vi "关键参数区.vi"(11 "数组":u16[](array[numeric]) format="%04xH") -> (3 "关键参数区":T1)   [LabVIEW 2016, in "CODCr库.lvlib"]
panel:
  # "共占用56 WORD"
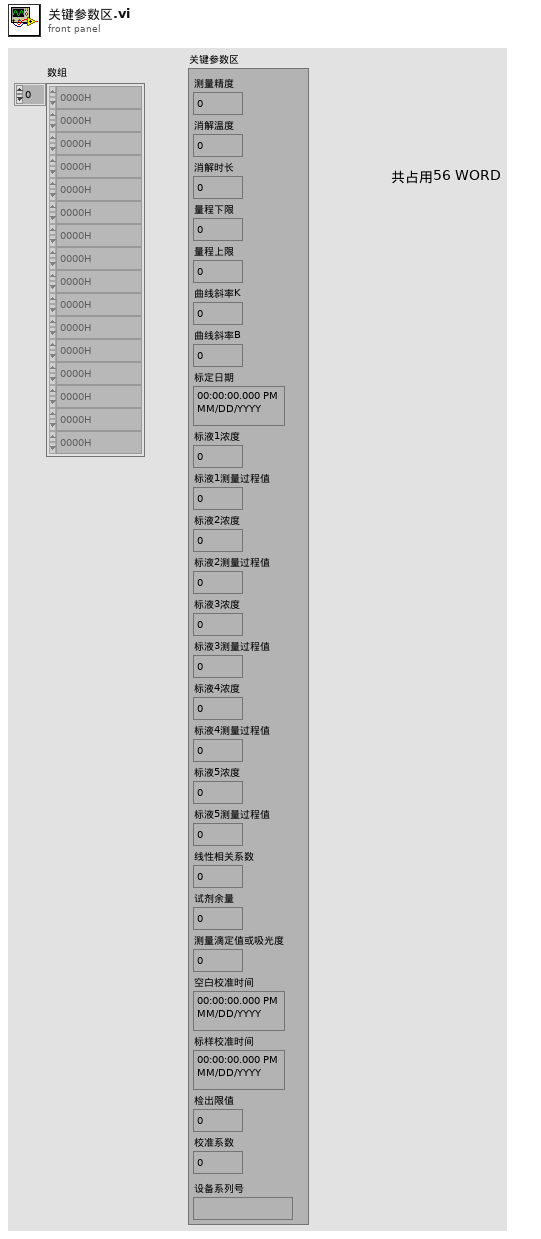
[diagram p1: front panel]
types:
  T1 = cluster{"测量精度":u16, "消解温度":u16, "消解时长":u16, "量程下限":sgl, "量程上限":sgl, "曲线斜率K":sgl, "曲线斜率B":sgl, "标定日期":timestamp, "标液1浓度":sgl, "标液1测量过程值":sgl, "标液2浓度":sgl, "标液2测量过程值":sgl, "标液3浓度":sgl, "标液3测量过程值":sgl, "标液4浓度":sgl, "标液4测量过程值":sgl, "标液5浓度":sgl, "标液5测量过程值":sgl, "线性相关系数":sgl, "试剂余量":u32, "测量滴定值或吸光度":sgl, "空白校准时间":timestamp, "标样校准时间":timestamp, "检出限值":sgl, "校准系数":sgl, "设备系列号":string}
  T2 = cluster{"WORD":u16, "WORD":u16, "WORD":u16, "FLOAT":sgl, "FLOAT":sgl, "FLOAT":sgl, "FLOAT":sgl, "time stamp":timestamp, "FLOAT":sgl, "FLOAT":sgl, "FLOAT":sgl, "FLOAT":sgl, "FLOAT":sgl, "FLOAT":sgl, "FLOAT":sgl, "FLOAT":sgl, "FLOAT":sgl, "FLOAT":sgl, "FLOAT":sgl, "DWORD":i32, "FLOAT":sgl, "time stamp":timestamp, "time stamp":timestamp, "FLOAT":sgl, "FLOAT":sgl, "string":string}
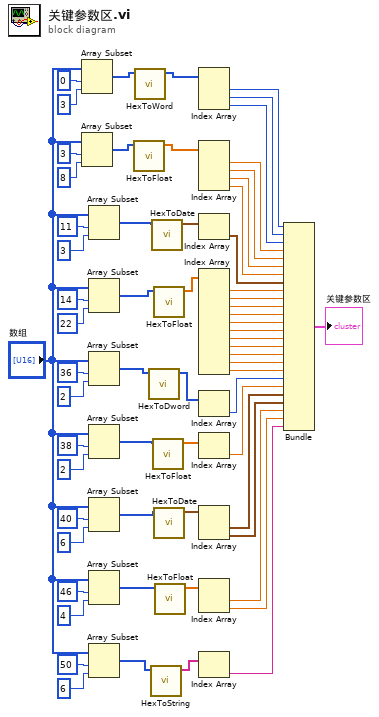
[diagram p0: block diagram]
diagram:
  n1 = Array Subset(array="数组", index=0 ("索引"), length=3 ("长度")) -> (w18:u16[])
  n2 = Array Subset(array="数组", index=3 ("索引"), length=8 ("长度")) -> (w15:u16[])
  n3 = Array Subset(array="数组", index=11 ("索引"), length=3 ("长度")) -> (w14:u16[])
  n4 = Array Subset(array="数组", index=14 ("索引"), length=22 ("长度")) -> (w11:u16[])
  n5 = Array Subset(array="数组", index=36 ("索引"), length=2 ("长度")) -> (w10:u16[])
  n6 = Array Subset(array="数组", index=38 ("索引"), length=2 ("长度")) -> (w8:u16[])
  n7 = Array Subset(array="数组", index=40 ("索引"), length=6 ("长度")) -> (w5:u16[])
  n8 = Array Subset(array="数组", index=46 ("索引"), length=4 ("长度")) -> (w3:u16[])
  n9 = Array Subset(array="数组", index=50 ("索引"), length=6 ("长度")) -> (w2:u16[])
  n10 = call "HexToFloat.vi"("数组"=w15) -> ("FLOAT"=w16:sgl[])  [unwired: 10 in]
  n11 = call "HexToWord.vi"("数组"=w18) -> ("WORD"=w17:u16[])  [unwired: 10 in]
  n12 = call "HexToDword.vi"("数组"=w10) -> ("DWORD"=w9:i32[])  [unwired: 10 in]
  n13 = call "HexToString.vi"("数组"=w2) -> ("STRING"=w1:string[])  [unwired: 10 in]
  n14 = call "HexToDate.vi"("数组"=w14) -> ("DATE"=w13:timestamp[])  [unwired: 10 in]
  n15 = call "HexToFloat.vi"("数组"=w8) -> ("FLOAT"=w7:sgl[])  [unwired: 10 in]
  n16 = call "HexToFloat.vi"("数组"=w11) -> ("FLOAT"=w12:sgl[])  [unwired: 10 in]
  n17 = call "HexToDate.vi"("数组"=w5) -> ("DATE"=w6:timestamp[])  [unwired: 10 in]
  n18 = call "HexToFloat.vi"("数组"=w3) -> ("FLOAT"=w4:sgl[])  [unwired: 10 in]
  n19 = Index Array(array=w17) -> (element #1=w62:u16, element #2=w61:u16, element #3=w60:u16)  [unwired: 3 in]
  n20 = Index Array(array=w16) -> (element #1=w57:sgl, element #2=w56:sgl, element #3=w55:sgl, element #4=w54:sgl)  [unwired: 4 in]
  n21 = Index Array(array=w13) -> (element=w51:timestamp)  [unwired: 1 in]
  n22 = Index Array(array=w12) -> (element #1=w48:sgl, element #2=w47:sgl, element #3=w46:sgl, element #4=w45:sgl, element #5=w27:sgl, element #6=w26:sgl, element #7=w25:sgl, element #8=w24:sgl, element #9=w23:sgl, element #10=w22:sgl, element #11=w21:sgl)  [unwired: 11 in]
  n23 = Index Array(array=w9) -> (element=w42:i32)  [unwired: 1 in]
  n24 = Index Array(array=w7) -> (element=w29:sgl)  [unwired: 1 in]
  n25 = Index Array(array=w6) -> (element #1=w39:timestamp, element #2=w38:timestamp)  [unwired: 2 in]
  n26 = Index Array(array=w4) -> (element #1=w35:sgl, element #2=w28:sgl)  [unwired: 2 in]
  n27 = Index Array(array=w1) -> (element=w19:string)  [unwired: 1 in]
  n28 = Bundle("WORD"=w62, "WORD"=w61, "WORD"=w60, "FLOAT"=w57, "FLOAT"=w56, "FLOAT"=w55, "FLOAT"=w54, "time stamp"=w51, "FLOAT"=w48, "FLOAT"=w47, "FLOAT"=w46, "FLOAT"=w45, "FLOAT"=w27, "FLOAT"=w26, "FLOAT"=w25, "FLOAT"=w24, "FLOAT"=w23, "FLOAT"=w22, "FLOAT"=w21, "DWORD"=w42, "FLOAT"=w29, "time stamp"=w39, "time stamp"=w38, "FLOAT"=w35, "FLOAT"=w28, "string"=w19) -> (→"关键参数区":T2)  [unwired: 1 in]
